vi "Initialize Rotate Close Thor WP.vi"() -> ()   [LabVIEW 2015]
uses:
  <vilib>/Utility/file.llb/Read From Spreadsheet File (DBL).vi
panel:
  out "WP zeros":dbl[](array[numeric])
  in  "Motion settings":path=path "C:/Users/SID4/Desktop/Joe Labview/SDT/Rotation Stages/Thorlabs APT/alicewpsetts190717.txt"
  in  "Rotate WP?":bool
  in  "MG17Motor 6":refnum<k7>(container)
  in  "MG17Motor 5":refnum<k7>(container)
  in  "MG17Motor 4":refnum<k7>(container)
  in  "MG17Motor 3":refnum<k7>(container)
  in  "MG17Motor 2":refnum<k7>(container)
  in  "MG17Motor":refnum<k7>(container)
  in  "stop":bool
  out "error out":errorcluster
  in  "error in (no error)":errorcluster
  in  "WP Vals":dbl[](array[numeric])=[0.0, 0.0, 0.0, 0.0, 0.0, 0.0]
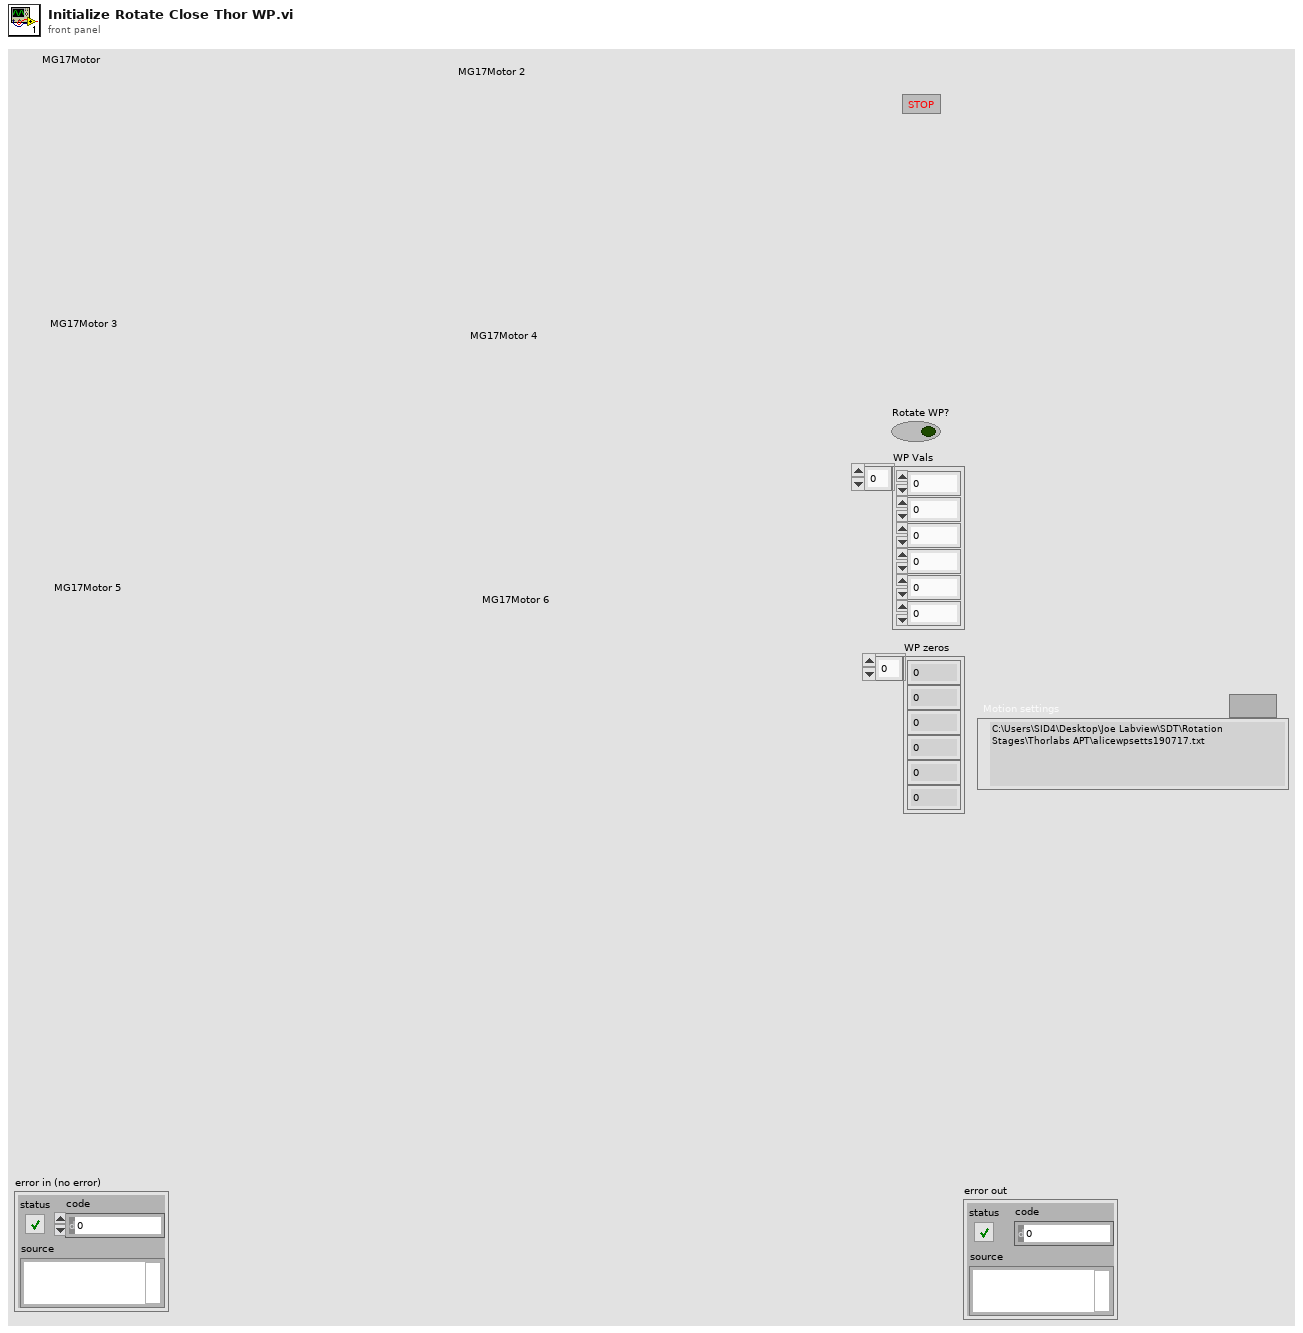
[diagram p1: front panel]
types:
  T1 = cluster{"MG17Motor":refnum<k7>, "MG17Motor 2":refnum<k7>, "MG17Motor 3":refnum<k7>, "MG17Motor 4":refnum<k7>, "MG17Motor 5":refnum<k7>, "MG17Motor 6":refnum<k7>}
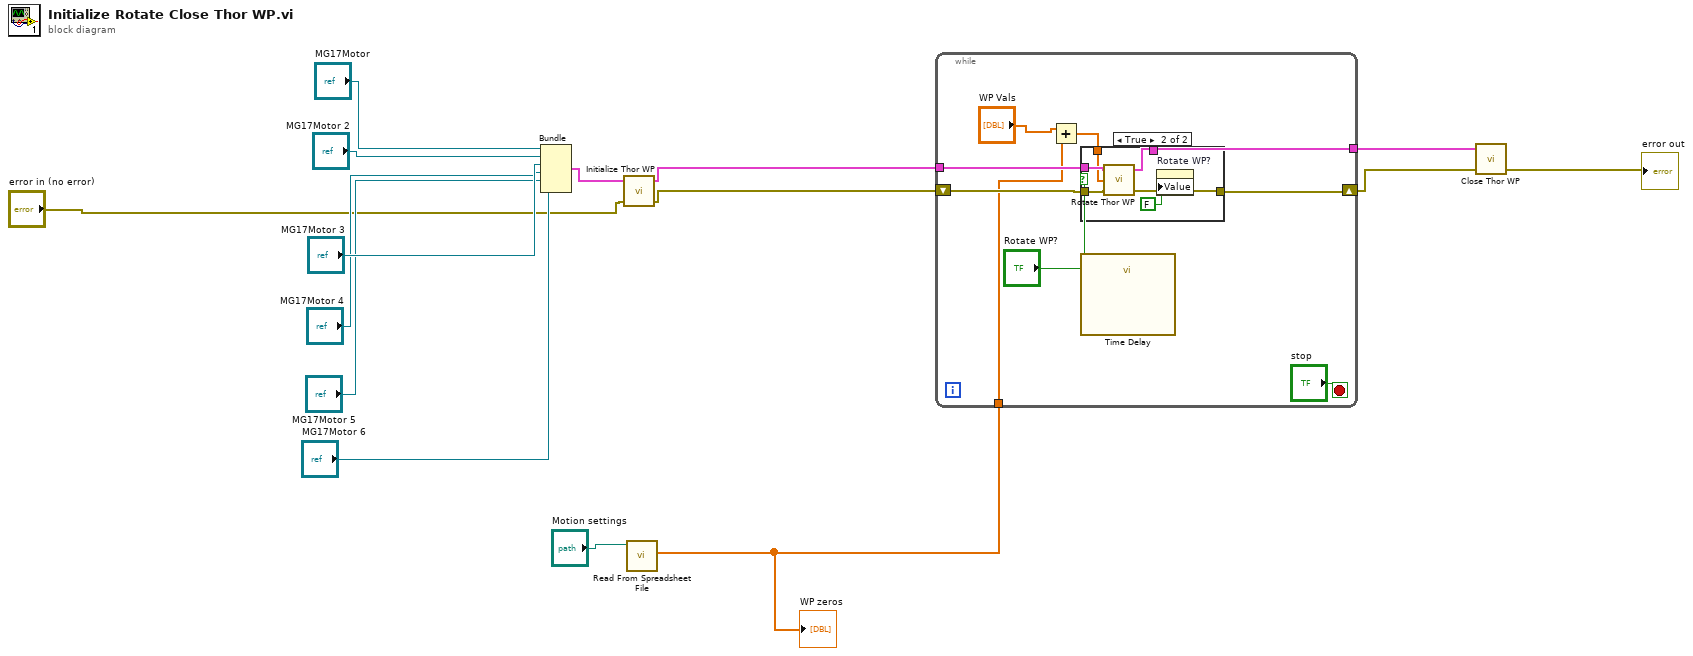
[diagram p0: block diagram]
diagram:
  n1 = Bundle("MG17Motor"="MG17Motor", "MG17Motor 2"="MG17Motor 2", "MG17Motor 3"="MG17Motor 3", "MG17Motor 4"="MG17Motor 4", "MG17Motor 5"="MG17Motor 5", "MG17Motor 6"="MG17Motor 6") -> (w8:T1)  [unwired: 1 in]
  n2 = call "Initialize Thor WP.vi"("error in (no error)"="error in (no error)", "input Kcube refnum cluster"=w8) -> ("error out"=w6:errorcluster, "output Kcube cluster"=w7:T1)  [unwired: 2 in]
  n3 = call-poly <vilib>:"Read From Spreadsheet File.vi"("file path (dialog if empty)"="Motion settings") -> ("first row"=w1:dbl[])  [unwired: 6 in, 4 out]
  "WP zeros" <- w1
  n4 = while {
    shift-right: [w22] -> w4
    shift-left: w6 -> [w23]
    tunnel: w7 -> [w21]
    tunnel: [w20] -> w5
    tunnel: w1 -> [w16]
    stop <- "stop" stop-if-true
    n5 = Add(x="WP Vals", y=w16) -> (x+y=w18:dbl[])
    n6 = case shown="True" "Rotate WP?" {
      tunnel: w23 -> [w25 w32]
      tunnel: [w25 w28] -> w22
      tunnel: w21 -> [w26 w31]
      tunnel: [w26 w30] -> w20
      tunnel: w18 -> [_ w29]
      frame False {
      }
      frame True {
        n7 = call "Rotate Thor WP.vi"("error in (no error)"=w32, "WP Vals"=w29, "input Kcube refnum cluster"=w31) -> ("error out"=w28:errorcluster, "output Kcube cluster"=w30:T1)  [unwired: 1 out]
        n8 = property on="Rotate WP?" class="Bool (strict)"("Value"=FALSE ("Rotate WP?")) -> ()  [unwired: 2 in, 2 out]
      }
    }
    n9 = call "Time Delay"() -> ()  [unwired: 11 in, 1 out]
  }
  n10 = call "Close Thor WP.vi"("error in (no error)"=w4, "input Kcube refnum cluster"=w5) -> ("error out"=→"error out":errorcluster)  [unwired: 3 in]
